vi "GreyRings.vi"(8 "error in (no error)":errorcluster, 11 "MAUI in":refnum<class "MAUI.lvclass">) -> (0 "error out":errorcluster, 3 "MAUI out":refnum<class "MAUI.lvclass">)   [LabVIEW 2019, in "MAUI.lvclass"]
uses:
  MAUI.lvclass
  MAUI.lvclass/MAUI.ctl
  34e12639-7869-429a-83b0-45689c5df1bf.vi
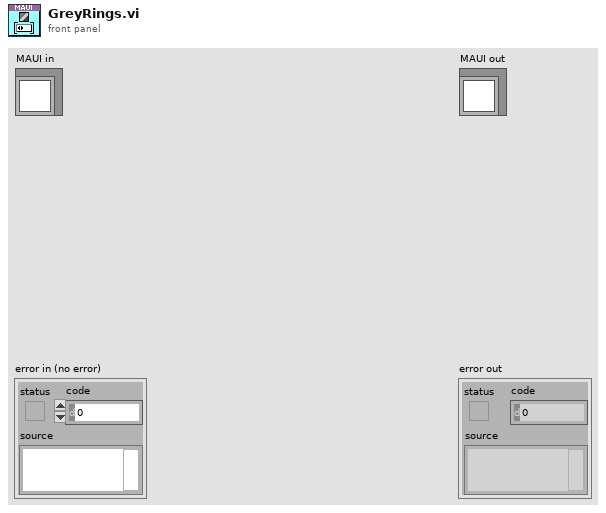
[diagram p1: front panel]
types:
  T1 = typedef "MAUI.lvclass/PanelData.ctl" = cluster{"SubPanel":refnum<vi>, "Ring":refnum<vi>, "Active":i32}
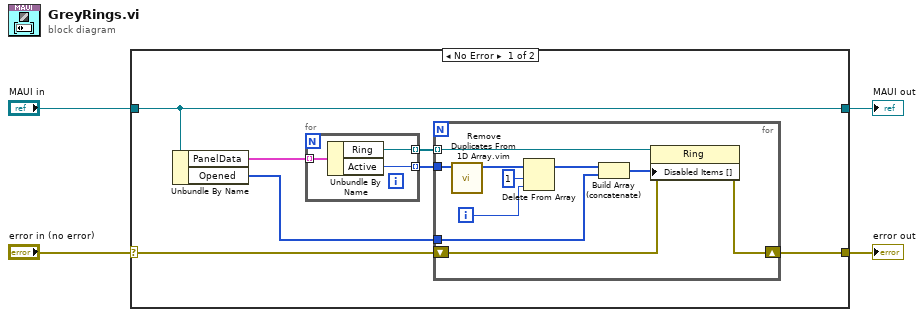
[diagram p0: block diagram]
diagram:
  n1 = case shown="No Error" "error in (no error)" {
    selector: "error in (no error)" -> [w7 w26]
    tunnel: [w6 w26] -> w3
    tunnel: [w11 w25] -> w1
    tunnel: "MAUI in" -> [w11 w25]
    frame No Error {
      n2 = Unbundle By Name(w11) -> ("PanelData"=w10:T1[], "Opened"=w5:i32[])
      n3 = for {
        tunnel: w10 -> [w24] mode=indexing
        tunnel: [w23] -> w9 mode=indexing
        tunnel: [w22] -> w8 mode=indexing
        n4 = Unbundle By Name(w24) -> ("Ring"=w22:refnum<vi>, "Active"=w23:i32)
      }
      n5 = for {
        tunnel: w9 -> [w17]
        tunnel: w8 -> [w21] mode=indexing
        shift-right: [w18] -> w6
        shift-left: w7 -> [w19]
        tunnel: w5 -> [w13]
        i -> [w12]
        n6 = call "Remove Duplicates From 1D Array.vim"("array"=w17) -> ("array with duplicates removed"=w16:i32[])  [unwired: 10 in]
        n7 = Delete From Array(array=w16, length=1, index=w12) -> (array with subset deleted=w15:i32[])  [unwired: 1 out]
        n8 = Build Array (concatenate)(w15, w13) -> (w14:i32[])
        n9 = property class="Ring"(reference=w21, error in=w19, "Disabled Items []"=w14) -> (error out=w18:errorcluster)  [unwired: 1 out]
      }
    }
    frame Error {
    }
  }
  "error out" <- w3
  "MAUI out" <- w1
